vi "Pi-DAR %28Sub VI%29.vi"(11 "I2CDevRef":T1 {"Device Address" format="%.0x"}) -> (0 "Distance Output":i32)   [LabVIEW 2014]
uses:
  <vilib>/Rock Robotics/WPI/I2C/WPI_I2CDevRef.ctl
  <vilib>/Rock Robotics/SystemInterfaces/Typedef/FPGA_TypedefDigitalModule.ctl
  <vilib>/Rock Robotics/SystemInterfaces/i2clib/i2c_bus.ctl
panel:
  out "Data Out":u8[](array[numeric])
  # "Outputs"
  # "Run this in a loop of 20 ms in periodic tasks.  We\nhave had success running it in a loop up to 15 ms,\nbut after that the values returned all went to zero.\n\nThe output value should be filtered using a rolling\naverage or other filter.  We used a 7 measurement\nrolling average."
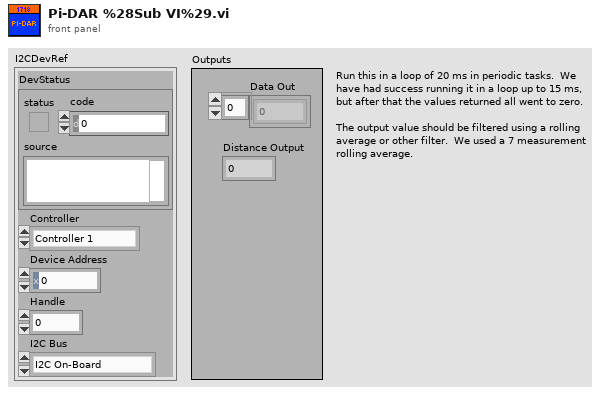
[diagram p1: front panel]
types:
  T1 = typedef "WPI_I2CDevRef.ctl" = cluster{"DevStatus":errorcluster, "Controller":T2, "Device Address":u8, "Handle":i32, "I2C Bus":T3}
  T2 = typedef "FPGA_TypedefDigitalModule.ctl" = enum16{"Controller 1"}
  T3 = typedef "i2c_bus.ctl" = enum16{"I2C On-Board", "I2C MXP", "Invalid"}
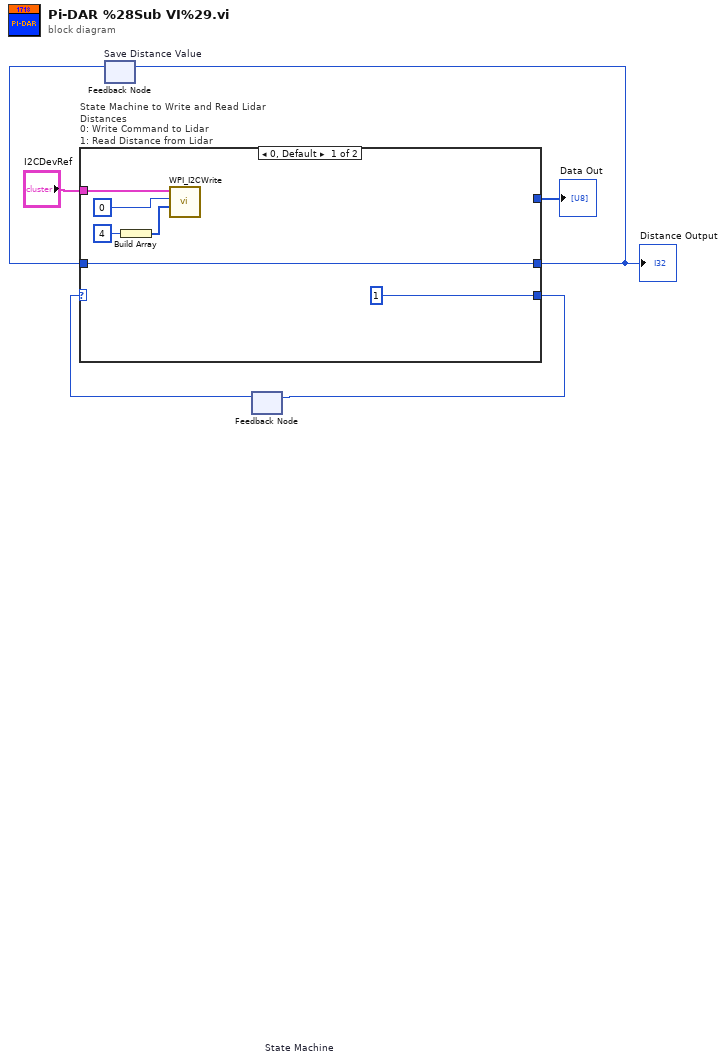
[diagram p0: block diagram]
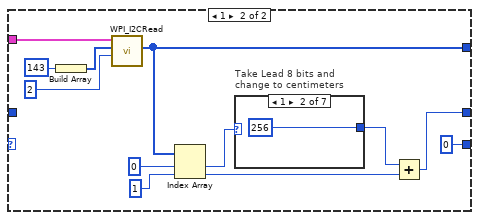
[diagram p2: hidden frame]
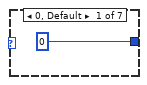
[diagram p3: hidden frame]
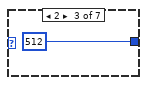
[diagram p4: hidden frame]
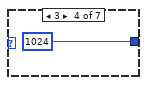
[diagram p5: hidden frame]
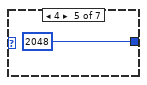
[diagram p6: hidden frame]
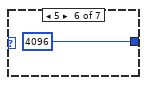
[diagram p7: hidden frame]
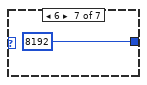
[diagram p8: hidden frame]
diagram:
  n1 = feedback #1 "Save Distance Value"() -> (w3:i32)  [unwired: 1 in]
  n2 = feedback #2 "State Machine"() -> (w5:i32)  [unwired: 1 in]
  n3 = case "State Machine to Write and Read Lidar Distances\n0: Write Command to Lidar\n1: Read Distance from Lidar" shown="0, Default" w5 {
    tunnel: "I2CDevRef" -> [w8 w24]
    tunnel: [1 0] -> w4
    tunnel: [w7 w14] -> w2
    tunnel: w3 -> [w7 _]
    tunnel: [_ w13] -> w6
    frame 0, Default {
      n4 = Build Array(u8 4 ("Data To Send")) -> (w11:u8[])
      n5 = call <vilib>:"WPI_I2CWrite.vi"("I2CDataToSend"=w11, "I2CRegister"=u8 0 ("Data To Send"), "I2CDevRef"=w8) -> ()  [unwired: 1 in, 8 out]
    }
    frame 1 {
      n6 = Build Array(u8 143 ("I2CRegister")) -> (w20:u8[])
      n7 = call <vilib>:"WPI_I2CRead.vi"("I2CBytesToRead"=u8 2, "I2CRegister"=w20, "I2CDevRef"=w24) -> ("Data Out"=w13:u8[])  [unwired: 6 in, 2 out]
      n8 = Index Array(array=w13, index #1=0 ("index"), index #2=1 ("index")) -> (element #1=w17:u8, element #2=w16:u8)
      n9 = case "Take Lead 8 bits and\nchange to centimeters" shown="1" w17 {
        tunnel: [0 256 512 1024 2048 4096 8192] -> w15
        frame 0, Default {
        }
        frame 1 {
        }
        frame 2 {
        }
        frame 3 {
        }
        frame 4 {
        }
        frame 5 {
        }
        frame 6 {
        }
      }
      n10 = Add(x=w15, y=w16) -> (x+y=w14:i32)
    }
  }
  "Data Out" <- w6
  "Distance Output" <- w2
  n11 = feedback-in #1(w2) -> ()
  n12 = feedback-in #2(w4) -> ()
